vi "Multiple Chassis Synchronization - Scopes Synchronized with TCLK.vi"() -> ()   [LabVIEW 2026]
uses:
  SubVIs/NI SYNC Abstraction/Lib/Trigger Routing.ctl
  SubVIs/NI SYNC Abstraction/Lib/Clock Routing.ctl
  <instrlib>/niScope/Controls/niScope export destinations.ctl
  Types/State.WithTclk.ctl
  <instrlib>/niScope/Controls/niScope input clock source.ctl
  Types/MyVariables.ctl
  <instrlib>/niScope/Controls/niScope exportable signals.ctl
  <instrlib>/niFgen/niFgen.llb/niFgen Output Mode.ctl
  <instrlib>/niScope/Configure/Trigger/niScope Configure Trigger Edge.vi
  <instrlib>/niScope/Configure/Trigger/niScope Configure Trigger Digital.vi
  SubVIs/NI SYNC Abstraction/Lib/Connect Clock Terminals-Array.vi
  SubVIs/NI SYNC Abstraction/Lib/Connect Clock Terminals.vi
  SubVIs/NI SYNC Abstraction/Lib/Connect Trigger Terminals.vi
  SubVIs/NI SYNC Abstraction/Lib/Disonnect Trigger Terminals-Array.vi
  SubVIs/NI SYNC Abstraction/Lib/Disonnect Trigger Terminals.vi
  <instrlib>/niScope/Acquire/Fetch/niScope Fetch Cluster.vi
  SubVIs/NI SYNC Abstraction/Lib/Disconnect Clock Terminals-Array.vi
  SubVIs/NI SYNC Abstraction/Lib/Disconnect Clock Terminals.vi
  <resource>/objmgr/sessionReference.rc
  <vilib>/ptbypt/NI_PtbyPt.lvlib
  <instrlib>/niSync/niSync.llb/niSync Initialize (IVI).vi
  SubVIs/NI SYNC Abstraction/Lib/Connect Trigger Terminals-Array.vi
panel:
  in  "Tab Control":T1(tab)
  in  "Master.Scope":refnum<k15>="PXI1_SCOPE1"
  in  "Rest.Scopes":refnum<k15>[](array[refnum])=["PXI2_SCOPE2"]
  in  "Master.6674T_1":refnum<k15>="PXI1_MasterSync"
  in  "Rest.6674T_1":refnum<k15>="PXI2_RestSync"
  in  "FGEN.Ref":refnum<k15>="PXI1_FGEN1"
  in  "Routing":T2(tab)
  in  "Rest.In --> Clk10":T3={"Source Terminal"="ClkIn", "Destination Terminal"="PXI_Clk10_In"}
  in  "Master.In --> Clk10":T3={"Source Terminal"="ClkIn", "Destination Terminal"="PXI_Clk10_In"}
  in  "Master.Clock --> Out":T3={"Source Terminal"="Oscillator", "Destination Terminal"="ClkOut"}
  in  "Rest.PFI --> Ref Trigger":T4={"Source"="PFI0", "Destination"="PXI_Trig0", "Synchronization Clock"="SyncClkAsync"}
  in  "Master.Ref Trigger --> PFI":T4={"Source"="PXI_Trig0", "Destination"="PFI0", "Synchronization Clock"="SyncClkAsync"}
  in  "Master.Ref Trigger Export":T5="VAL_RTSI_0"
  in  "Rest.Ref Trigger Source":T5="VAL_RTSI_0"
  in  "Rest.Start Trigger Source":T5="VAL_RTSI_1"
  in  "Rest.PFI --> Start Trigger":T4={"Source"="PFI1", "Destination"="PXI_Trig1", "Synchronization Clock"="SyncClkAsync"}
  in  "Master.Start Trigger --> PFI":T4={"Source"="PXI_Trig1", "Destination"="PFI2", "Synchronization Clock"="SyncClkAsync"}
  in  "Master.Start Trigger Export":T5="VAL_RTSI_1"
  in  "Rest.Sync Pulse Source":string(combo)="PXI_Trig2"
  in  "Rest.PFI --> Sync Pulse Source":T4={"Source"="PFI1", "Destination"="PXI_Trig2", "Synchronization Clock"="SyncClkAsync"}
  in  "Master.PFI --> Sync Pulse Source":T4={"Source"="PFI1", "Destination"="PXI_Trig2", "Synchronization Clock"="SyncClkAsync"}
  in  "Master.Sync Pulse Export --> PFI":T4={"Source"="PXI_Trig3", "Destination"="PFI2", "Synchronization Clock"="SyncClkFullSpeed"}
  in  "Master.Sync Pulse Export":string(combo)="PXI_Trig3"
  in  "Master.Sync Pulse Source":string(combo)="PXI_Trig2"
  in  "Enable Cal?":bool
  in  "Calibration Iterations":i32=10
  in  "Master Scope tCLK Delay":dbl format="%#_13p"
  out "Cal Iteration Delays":dbl[](array[numeric]) format="%#_p"
  out "Average Delay":dbl format="%.5p"
  out "Standard Deviation":dbl format="%0.2p"
  out "Waveform Graph":T6(graph)
  out "Sample Offset":dbl
  out "error out":errorcluster
  out "Offset Time (s)":dbl format="%#_p"
  # "Scope"
  # "Sync"
  # "Master"
  # "Ref Trigger Export"
  # "Start Trigger Export"
  # "Sync Pulse Source"
  # "Sync Pulse Export"
  # "Sync"
  # "Scope"
  # "Rest"
  # "Ref Trigger Source"
  # "Start Trigger Source"
  # "Sync Pulse Source"
  # "None"
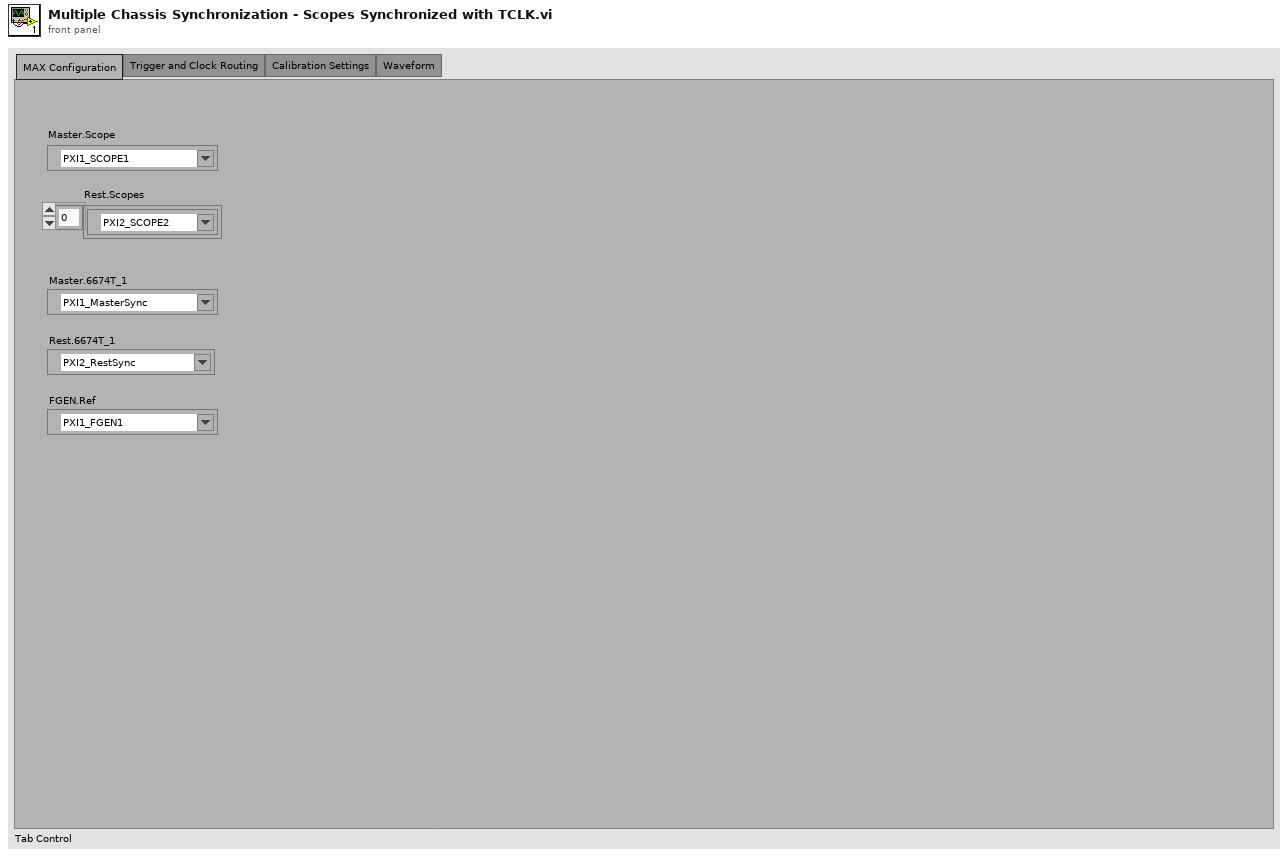
[diagram p1: front panel]
types:
  T1 = enum32{"MAX Configuration", "Trigger and Clock Routing", "Calibration Settings", "Waveform"}
  T2 = enum32{"Clock Routing", "Reference Trigger", "Start Trigger", "Sync Pulse"}
  T3 = typedef "Clock Routing.ctl" = cluster{"Source Terminal":string, "Destination Terminal":string}
  T4 = typedef "Trigger Routing.ctl" = cluster{"Source":string, "Destination":string, "Synchronization Clock":string}
  T5 = typedef "niScope export destinations.ctl" = string
  T6 = cluster{"relativeInitialX":dbl, "xIncrement":dbl, "wfm":dbl[]}[]
  T7 = typedef "State.WithTclk.ctl" = enum16{"Initialize", "SCOPE: Config.Master", "SCOPE: Config.Rest", "SYNC: Device.Init", "SYNC: ConnectClock.Master", "SYNC: ConnectClock.Rest", "SYNC: ConnectSyncPulse.Master", "SYNC: ConnectSyncPulse.Rest", "SYNC: ConnectRefTrigger.Master", "SYNC: ConnectRefTrigger.Rest", "TCLK: Config.Master", "TCLK: Config.Rest", "TCLK: ApplyManualCalibration", "TCLK: SendSyncPulse", "SYNC: DisconnectSyncPulse.Master", "SYNC: DisconnectSyncPulse.Rest", "SYNC: ConnectStartTrigger.Master", "SYNC: ConnectStartTrigger.Rest", "TCLK: Commit", "FGEN: StartSquareWave", "SCOPE: Acquire", "FGEN: StopSquareWave", "SYNC: DisconnectStartTrigger.Master", "SYNC: DisconnectStartTrigger.Rest", "SYNC: DisconnectRefTrigger.Master", "SYNC: DisconnectRefTrigger.Rest", "SYNC: DisconnectClock.Master", "SYNC: DisconnectClock.Rest", "Shutdown"}
  T8 = typedef "MyVariables.ctl" = cluster{"Master":cluster{"TimeSync.Ref":refnum<k15>, "TCLK.Ref":refnum<k20>, "Clock":cluster{"Clock --> Out":T3, "In --> Clk10":T3}, "Sync Pulse":cluster{"Sync Pulse Export":string, "Sync Pulse Export --> PFI":T4, "PFI --> Sync Pulse Source":T4, "Sync Pulse Source":string}, "Start Trigger":cluster{"Start Trigger Export":T5, "Start Trigger --> PFI":T4}, "Scope.Ref":refnum<k15>, "Ref Trigger":cluster{"Ref Trigger Export":T5, "Ref Trigger --> PFI":T4}}, "Rest":cluster{"TimeSync.Ref":refnum<k15>, "TCLK.Refs":refnum<k20>[], "Clock":cluster{"In --> Clk10":T3}, "Sync Pulse":cluster{"PFI --> Sync Pulse Source":T4, "Sync Pulse Source":string}, "Start Trigger":cluster{"PFI --> Start Trigger":T4, "Start Trigger Source":T5}, "Scope.Refs":refnum<k15>[], "Ref Trigger":cluster{"PFI --> Ref Trigger":T4, "Ref Trigger Source":T5}}, "FGEN.Ref":refnum<k15>}
  T9 = typedef "niScope input clock source.ctl" = u16
  T10 = typedef "niScope exportable signals.ctl" = u16
  T11 = typedef "niFgen Output Mode.ctl" = u32
  T12 = cluster{"relativeInitialX":dbl, "xIncrement":dbl, "wfm":dbl[]}
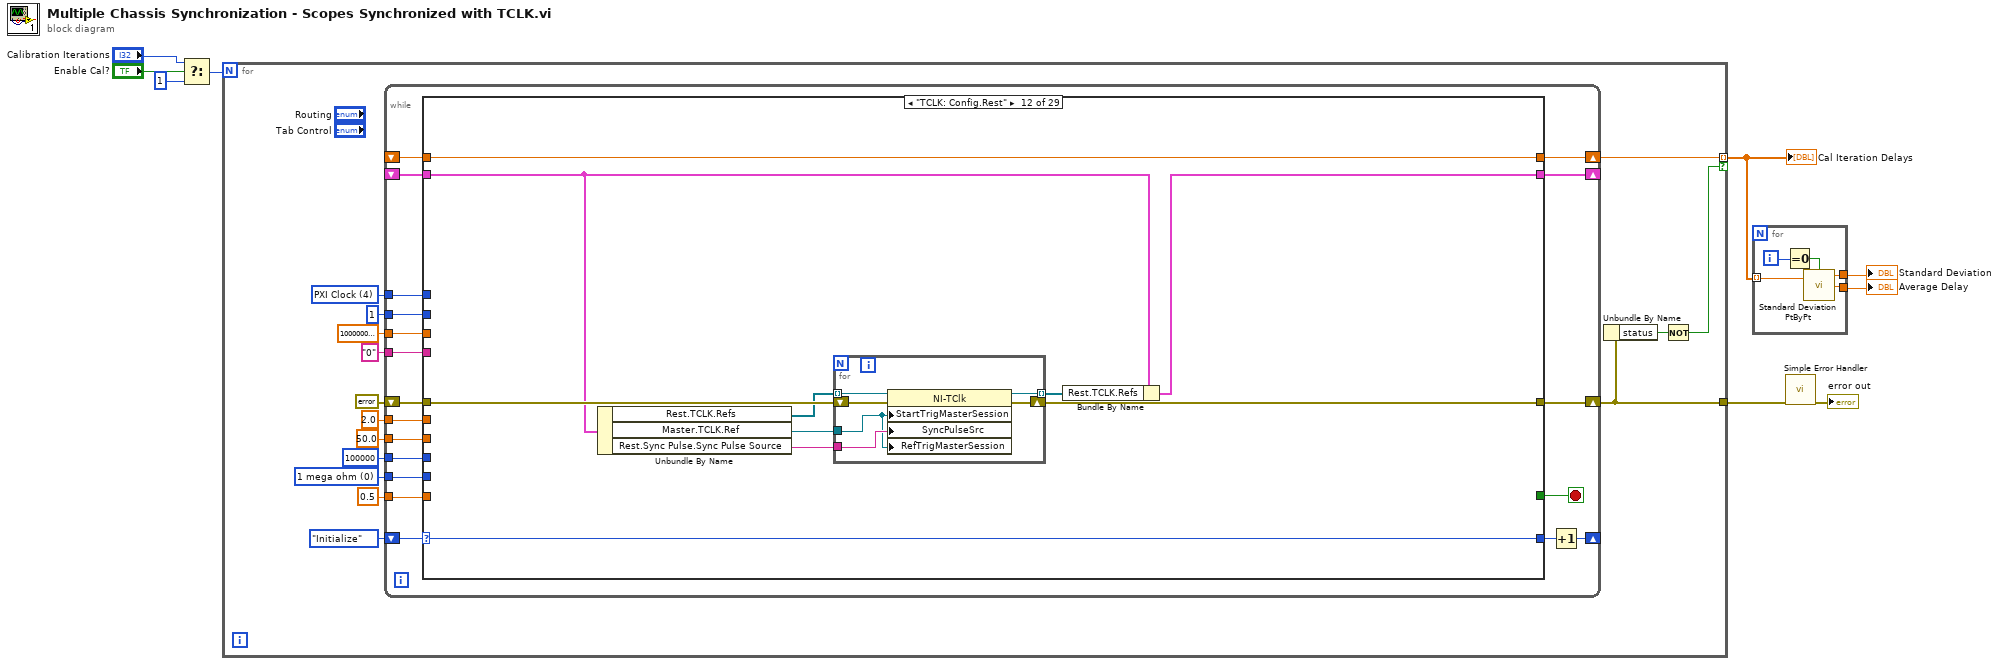
[diagram p0: block diagram]
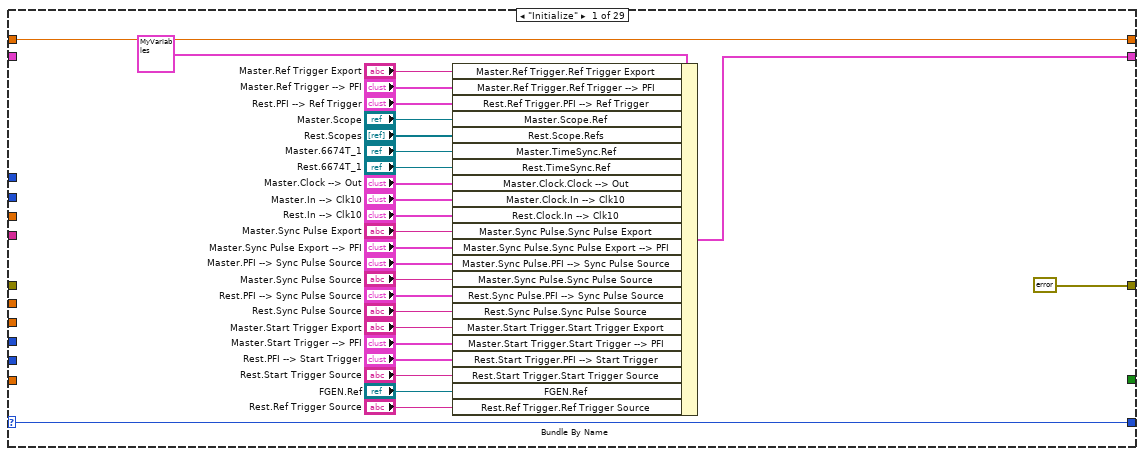
[diagram p2: hidden frame]
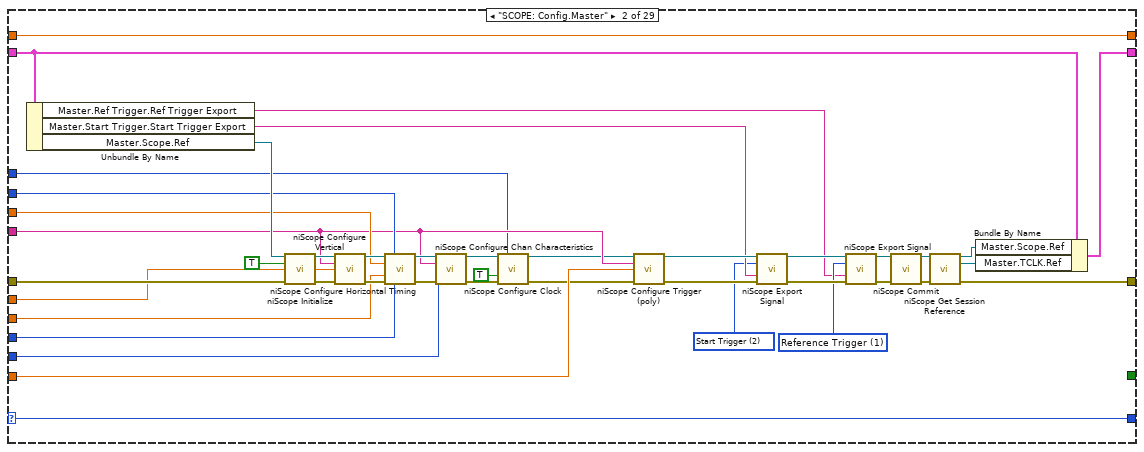
[diagram p3: hidden frame]
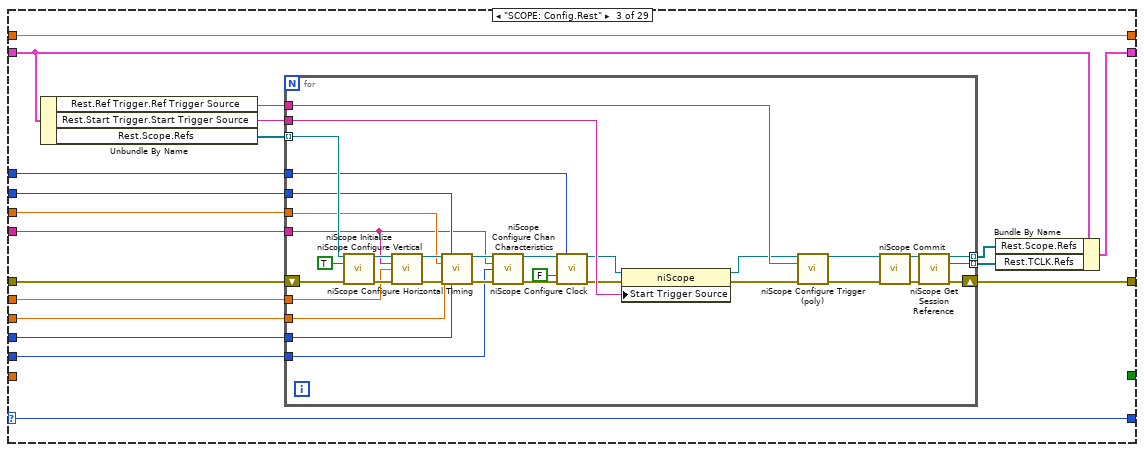
[diagram p4: hidden frame]
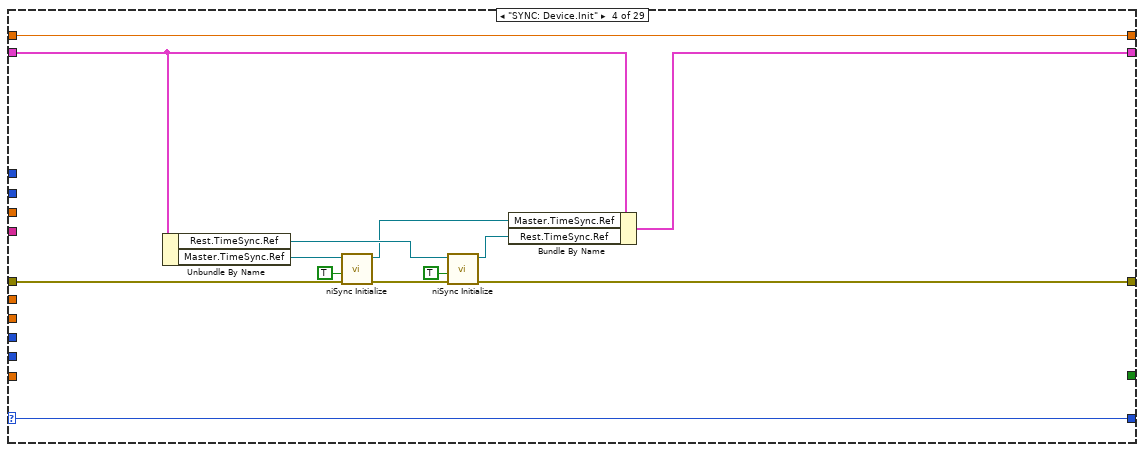
[diagram p5: hidden frame]
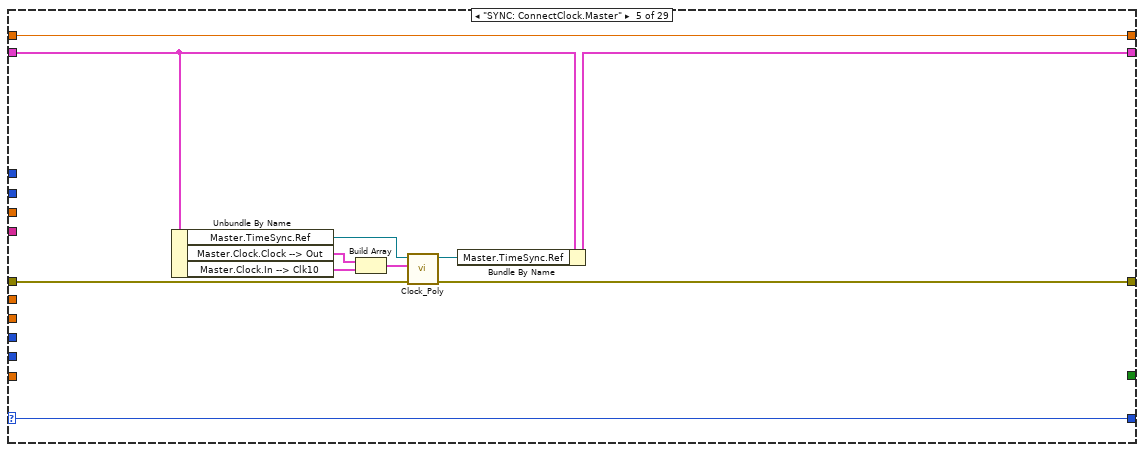
[diagram p6: hidden frame]
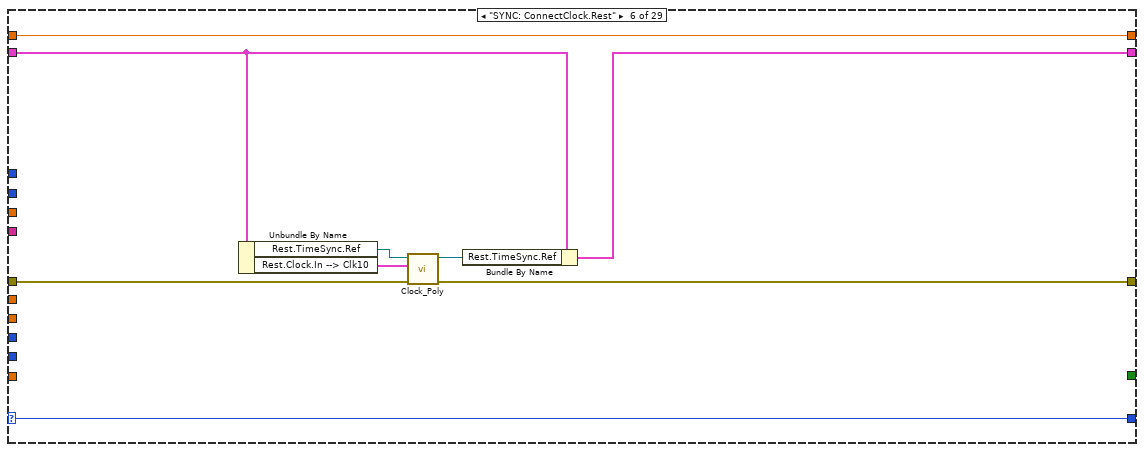
[diagram p7: hidden frame]
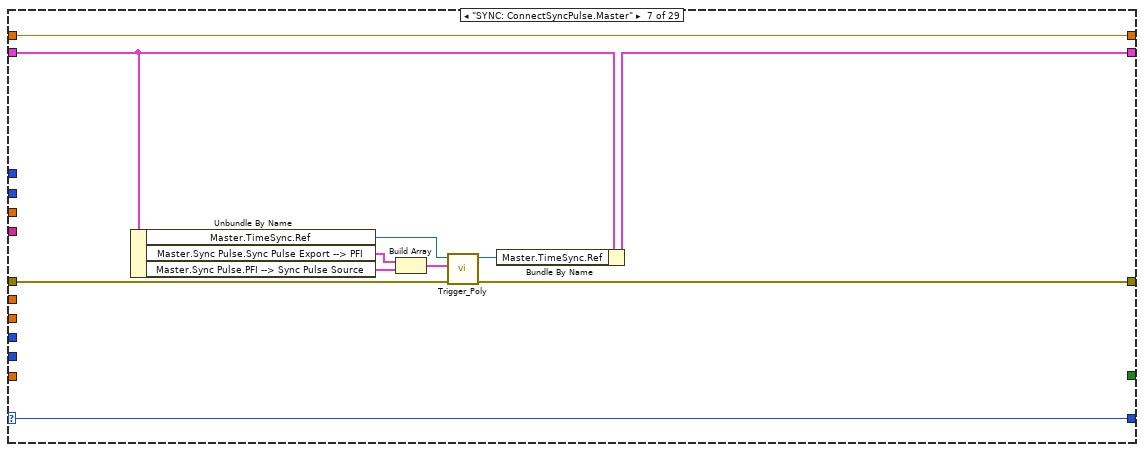
[diagram p8: hidden frame]
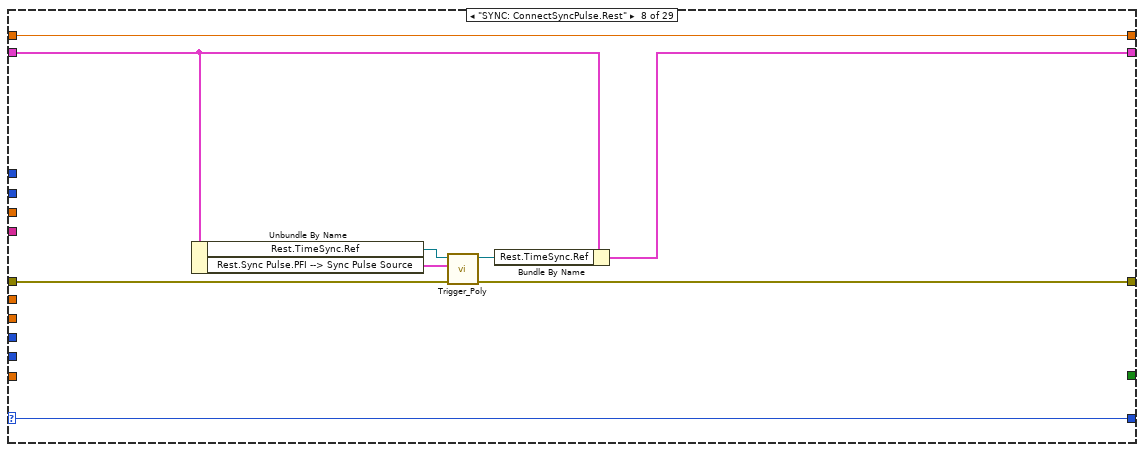
[diagram p9: hidden frame]
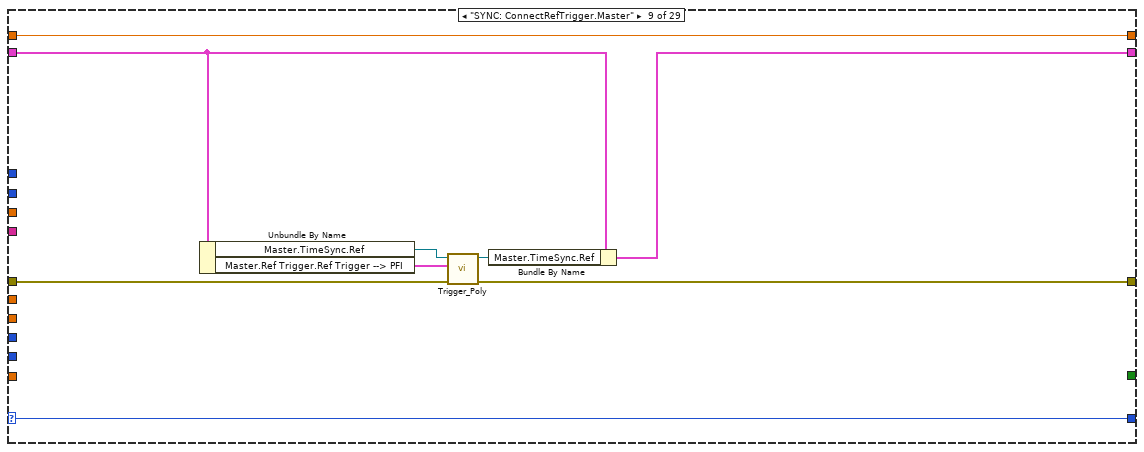
[diagram p10: hidden frame]
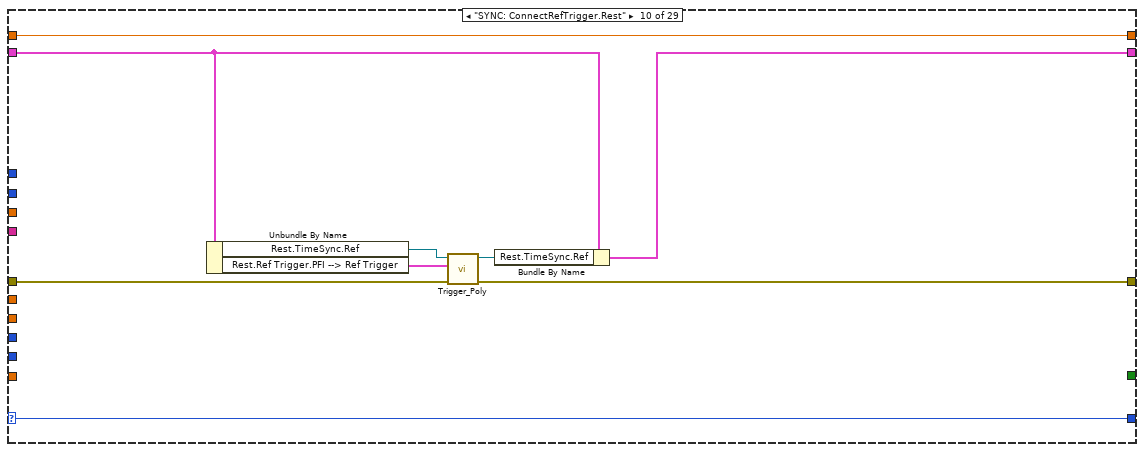
[diagram p11: hidden frame]
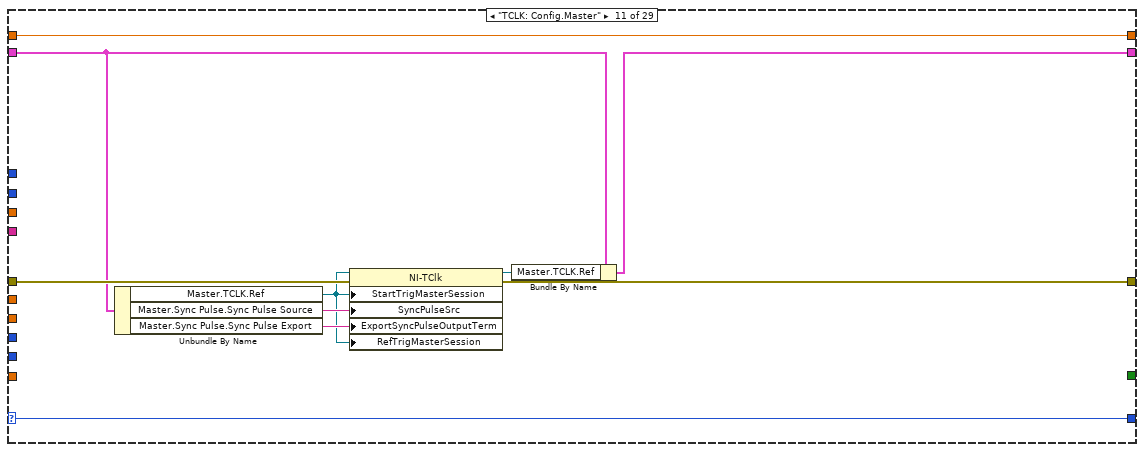
[diagram p12: hidden frame]
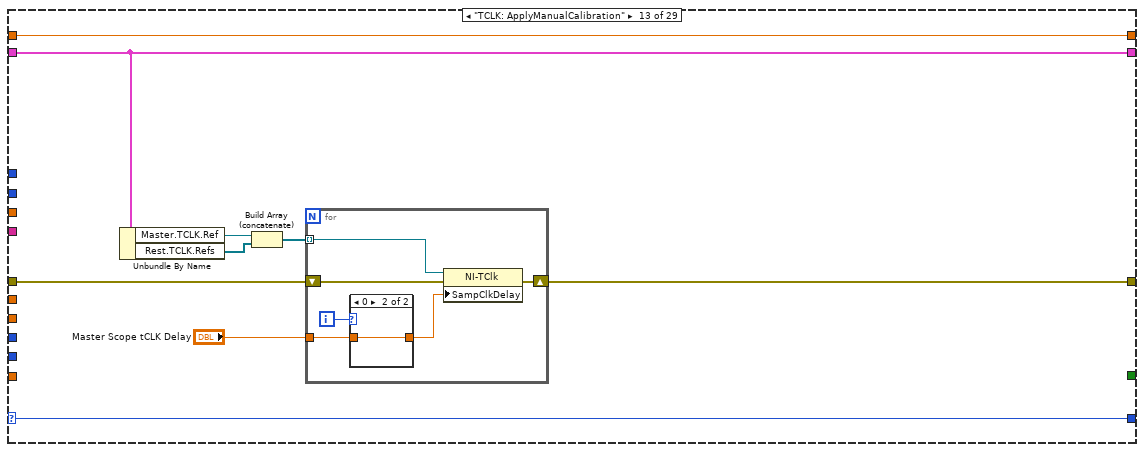
[diagram p13: hidden frame]
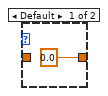
[diagram p14: hidden frame]
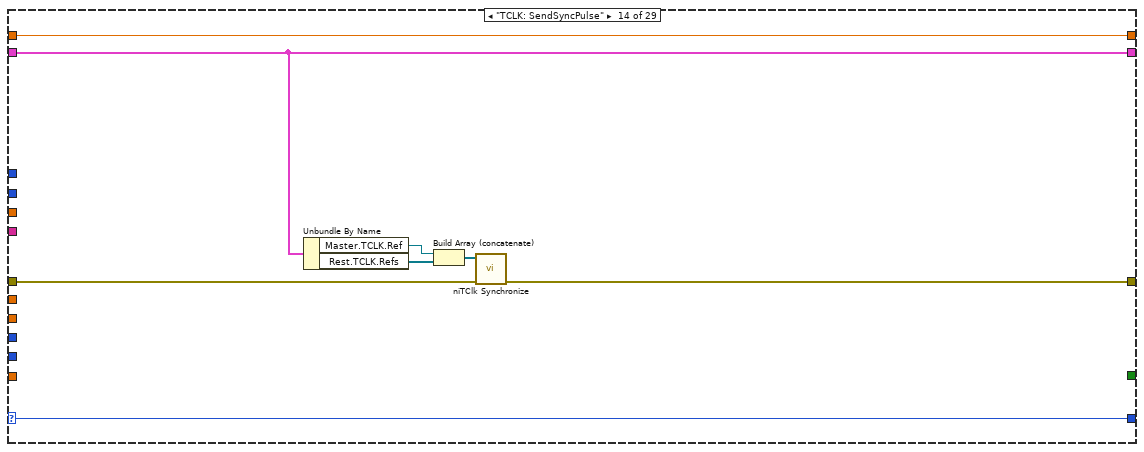
[diagram p15: hidden frame]
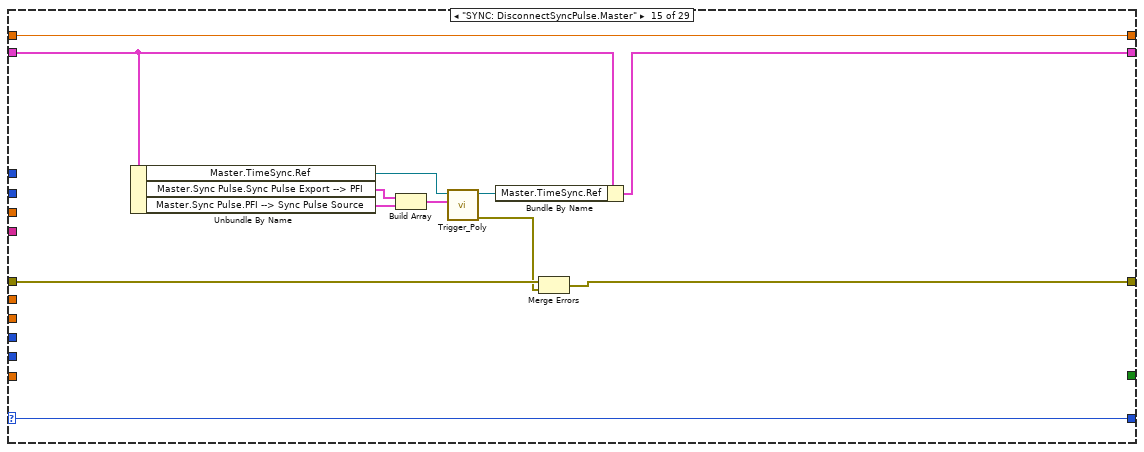
[diagram p16: hidden frame]
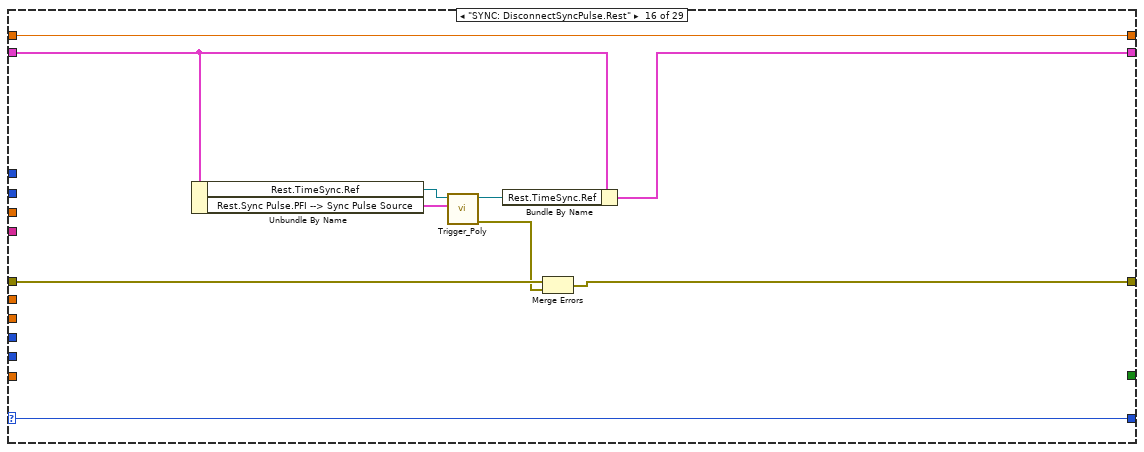
[diagram p17: hidden frame]
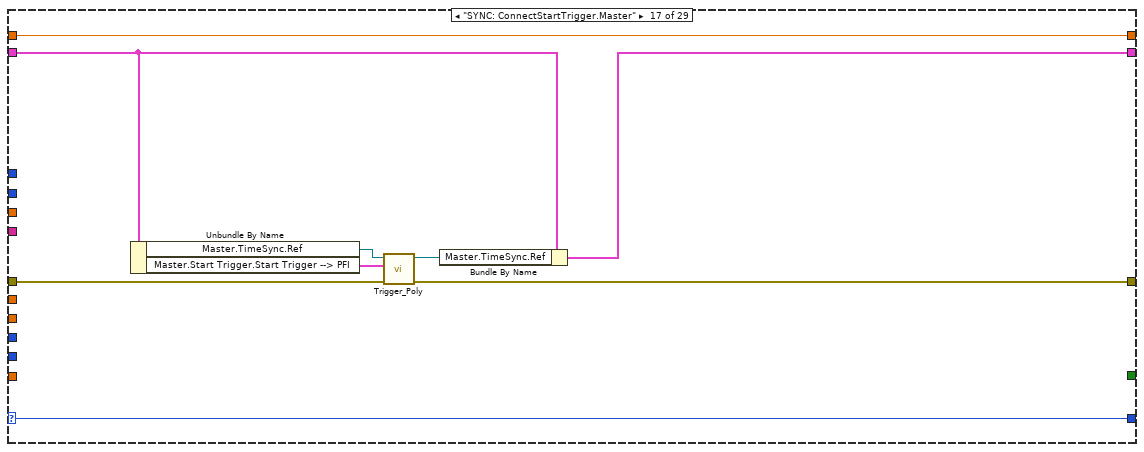
[diagram p18: hidden frame]
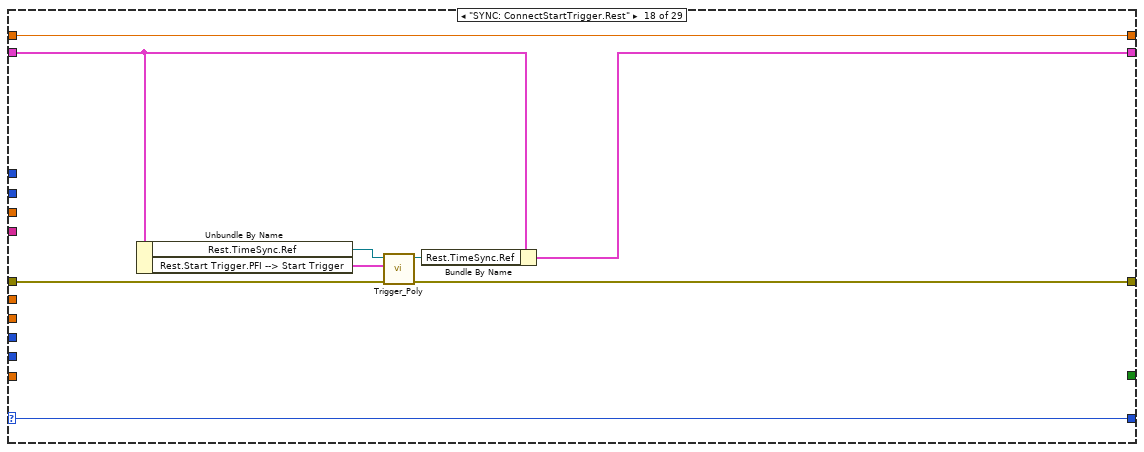
[diagram p19: hidden frame]
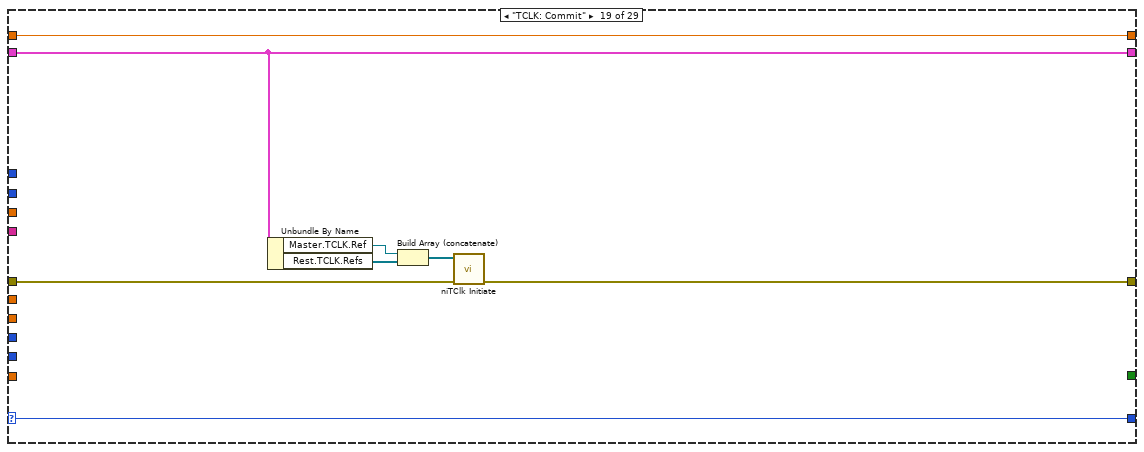
[diagram p20: hidden frame]
diagram:
  n1 = Select(t="Calibration Iterations", s="Enable Cal?", f=1) -> (s? t:f=w4:i32)
  n2 = for {
    N: w4 -> [_]
    tunnel: [w13] -> w9
    tunnel: [w14] -> w3 mode=indexing if=w11
    w10 = T9 4 items=["None"=0, "RTSI Clock"=1, "PFI 0"=6, "PFI 1"=2, "PFI 2"=3, "PXI Clock"=4, "External"=5, "Clock In"=7] ("input clock source")
    w18 = u32 0 items=["1 mega ohm"=0, "50 ohms"=2] ("input impedance")
    n3 = while {
      shift-right: [w36] -> _
      shift-left: State.WithTclk."Initialize" -> [w43]
      shift-right: [w42] -> _
      shift-left: _ -> [w41]
      shift-right: [w39] -> w13
      shift-left: errorcluster {"status"=FALSE, "code"=0, "source"=""} ("error out") -> [w40]
      tunnel: 100000000.0 ("min sample rate") -> [w35]
      tunnel: 100000 ("min record length") -> [w34]
      tunnel: 2.0 ("vertical offset") -> [w33]
      tunnel: 50.0 ("reference position") -> [w32]
      tunnel: w18 -> [w31]
      tunnel: 1 ("number of records") -> [w30]
      tunnel: "0" ("channels") -> [w29]
      tunnel: 0.5 ("trigger level") -> [w28]
      shift-right: [w27] -> w14
      shift-left: _ -> [w26]
      tunnel: w10 -> [w25]
      stop <- w37 stop-if-true
      n4 = case shown="\"TCLK: Config.Rest\"" w43 {
        selector: w43 -> [w53 w112 w131 w167 w179 w191 w199 w211 w220 w229 w245 w255 w270 w286 w291 w304 w311 w320 w334 w344 w376 w388 w400 w411 w421 w431 w440 w453 w460]
        tunnel: [w54 w110 w130 w171 w187 w196 w207 w216 w225 w234 w238 w248 w269 w283 w297 w307 w316 w325 w331 w342 w373 w393 w404 w414 w424 w434 w446 w456 w471] -> w42
        tunnel: w41 -> [_ w96 w127 w172 w188 w197 w208 w217 w226 w235 w240 w250 w269 w283 w298 w308 w317 w326 w331 w336 w373 w393 w405 w415 w425 w435 w447 w457 w471]
        tunnel: [w53 w112 w131 w167 w179 w191 w199 w211 w220 w229 w245 w255 w270 w286 w291 w304 w311 w320 w334 w344 w376 w388 w400 w411 w421 w431 w440 w453 w460] -> w38
        tunnel: [errorcluster {"status"=FALSE, "code"=0, "source"=""} ("error out") w109 w129 w168 w184 w193 w204 w213 w222 w231 w243 w253 w267 w284 w288 w300 w313 w322 w328 w345 w370 w389 w398 w409 w417 w428 w438 w450 w461] -> w39
        tunnel: w40 -> [_ w98 w128 w166 w180 w192 w200 w212 w221 w230 w244 w254 w268 w285 w290 w302 w312 w321 w329 w346 w375 w390 w397 w407 w419 w427 w439 w451 w464]
        tunnel: [_ _ _ _ _ _ _ _ _ _ _ _ _ _ _ _ _ _ _ _ _ _ _ _ _ _ _ _ TRUE] -> w37
        tunnel: w35 -> [_ w84 w120 _ _ _ _ _ _ _ _ _ _ _ _ _ _ _ _ _ w361 _ _ _ _ _ _ _ _]
        tunnel: w34 -> [_ w83 w116 _ _ _ _ _ _ _ _ _ _ _ _ _ _ _ _ _ w362 _ _ _ _ _ _ _ _]
        tunnel: w33 -> [_ w82 w118 _ _ _ _ _ _ _ _ _ _ _ _ _ _ _ _ _ _ _ _ _ _ _ _ _ _]
        tunnel: w32 -> [_ w81 w117 _ _ _ _ _ _ _ _ _ _ _ _ _ _ _ _ _ _ _ _ _ _ _ _ _ _]
        tunnel: w31 -> [_ w80 w115 _ _ _ _ _ _ _ _ _ _ _ _ _ _ _ _ _ _ _ _ _ _ _ _ _ _]
        tunnel: w30 -> [_ w79 w121 _ _ _ _ _ _ _ _ _ _ _ _ _ _ _ _ _ _ _ _ _ _ _ _ _ _]
        tunnel: w29 -> [_ w78 w119 _ _ _ _ _ _ _ _ _ _ _ _ _ _ _ _ _ _ _ _ _ _ _ _ _ _]
        tunnel: w28 -> [_ w77 _ _ _ _ _ _ _ _ _ _ _ _ _ _ _ _ _ w340 w358 _ _ _ _ _ _ _ _]
        tunnel: [w45 w76 w114 w165 w178 w189 w198 w209 w218 w227 w236 w246 w263 w279 w287 w299 w309 w318 w327 w337 w357 w387 w396 w406 w416 w426 w436 w448 w458] -> w27
        tunnel: w26 -> [w45 w76 w114 w165 w178 w189 w198 w209 w218 w227 w236 w246 w263 w279 w287 w299 w309 w318 w327 w337 _ w387 w396 w406 w416 w426 w436 w448 w458]
        tunnel: w25 -> [_ w72 w113 _ _ _ _ _ _ _ _ _ _ _ _ _ _ _ _ _ _ _ _ _ _ _ _ _ _]
        frame "Initialize" {
          n5 = Bundle By Name(cluster=T8 {"Master"={"TimeSync.Ref"="PXI_Trig0", "TCLK.Ref"=refnum, "Clock"={"Clock --> Out"={"Source Terminal"="Oscillator", "Destination Terminal"="ClkOut"}, "In --> Clk10"={"Source Terminal"="ClkIn", "Destination Terminal"="PXI_Clk10_In"}}, "Sync Pulse"={"Sync Pulse Export"="SyncClkFullSpeed", "Sync Pulse Export --> PFI"={"Source"="ClkIn", "Destination"="PXI_Clk10_In", "Synchronization Clock"="SyncClkAsync"}, "PFI --> Sync Pulse Source"={"Source"="PXI_Trig2", "Destination"="PFI2", "Synchronization Clock"="SyncClkAsync"}, "Sync Pulse Source"="PFI1"}, "Start Trigger"={"Start Trigger Export"="PXI_Trig2", "Start Trigger --> PFI"={"Source"="SyncClkAsync", "Destination"="VAL_RTSI_2", "Synchronization Clock"=""}}, "Scope.Ref"="", "Ref Trigger"={"Ref Trigger Export"="VAL_RTSI_2", "Ref Trigger --> PFI"={"Source"="PXI_Trig3", "Destination"="PFI0", "Synchronization Clock"="SyncClkAsync"}}}, "Rest"={"TimeSync.Ref"="", "TCLK.Refs"=[], "Clock"={"In --> Clk10"={"Source Terminal"="PXI_Trig0", "Destination Terminal"="PFI2"}}, "Sync Pulse"={"PFI --> Sync Pulse Source"={"Source"="PFI1", "Destination"="PXI_Trig1", "Synchronization Clock"="SyncClkAsync"}, "Sync Pulse Source"="PXI_Trig1"}, "Start Trigger"={"PFI --> Start Trigger"={"Source"="PFI1", "Destination"="PXI_Trig2", "Synchronization Clock"="SyncClkAsync"}, "Start Trigger Source"="VAL_RTSI_2"}, "Scope.Refs"=[], "Ref Trigger"={"PFI --> Ref Trigger"={"Source"="PFI0", "Destination"="PXI_Trig3", "Synchronization Clock"="SyncClkAsync"}, "Ref Trigger Source"="VAL_RTSI_3"}}, "FGEN.Ref"=""} ("Routes"), "Master.Ref Trigger.Ref Trigger Export"="Master.Ref Trigger Export", "Master.Ref Trigger.Ref Trigger --> PFI"="Master.Ref Trigger --> PFI", "Rest.Ref Trigger.PFI --> Ref Trigger"="Rest.PFI --> Ref Trigger", "Master.Scope.Ref"="Master.Scope", "Rest.Scope.Refs"="Rest.Scopes", "Master.TimeSync.Ref"="Master.6674T_1", "Rest.TimeSync.Ref"="Rest.6674T_1", "Master.Clock.Clock --> Out"="Master.Clock --> Out", "Master.Clock.In --> Clk10"="Master.In --> Clk10", "Rest.Clock.In --> Clk10"="Rest.In --> Clk10", "Master.Sync Pulse.Sync Pulse Export"="Master.Sync Pulse Export", "Master.Sync Pulse.Sync Pulse Export --> PFI"="Master.Sync Pulse Export --> PFI", "Master.Sync Pulse.PFI --> Sync Pulse Source"="Master.PFI --> Sync Pulse Source", "Master.Sync Pulse.Sync Pulse Source"="Master.Sync Pulse Source", "Rest.Sync Pulse.PFI --> Sync Pulse Source"="Rest.PFI --> Sync Pulse Source", "Rest.Sync Pulse.Sync Pulse Source"="Rest.Sync Pulse Source", "Master.Start Trigger.Start Trigger Export"="Master.Start Trigger Export", "Master.Start Trigger.Start Trigger --> PFI"="Master.Start Trigger --> PFI", "Rest.Start Trigger.PFI --> Start Trigger"="Rest.PFI --> Start Trigger", "Rest.Start Trigger.Start Trigger Source"="Rest.Start Trigger Source", "FGEN.Ref"="FGEN.Ref", "Rest.Ref Trigger.Ref Trigger Source"="Rest.Ref Trigger Source") -> (w54:T8)
        }
        frame "SCOPE: Config.Master" {
          w86 = T10 1 items=["None"=0, "Start Trigger"=2, "Advance Trigger"=5, "Reference Trigger"=1, "End of Record Event"=4, "End of Acquisition Event"=3, "Ready for Start Event"=7, "Ready for Advance Event"=6, "Ready for Reference Event"=10, "Reference Clock"=100, "Sample Clock"=101, "5 Volt Power"=13] ("signal")
          w91 = T10 2 items=["None"=0, "Start Trigger"=2, "Advance Trigger"=5, "Reference Trigger"=1, "End of Record Event"=4, "End of Acquisition Event"=3, "Ready for Start Event"=7, "Ready for Advance Event"=6, "Ready for Reference Event"=10, "Reference Clock"=100, "Sample Clock"=101, "5 Volt Power"=13] ("signal")
          n6 = Unbundle By Name(w96) -> ("Master.Ref Trigger.Ref Trigger Export"=w85:T5, "Master.Start Trigger.Start Trigger Export"=w95:T5, "Master.Scope.Ref"=w94:refnum<k15>)
          n7 = call <instrlib>:"niScope Initialize.vi"("resource name"=w94, "id query"=TRUE, "error in"=w98) -> ("instrument handle"=w107:refnum<k15>, "error out"=w104:errorcluster)  [unwired: 11 in]
          n8 = call <instrlib>:"niScope Configure Vertical.vi"("instrument handle"=w107, "channels"=w78, "vertical range"=w82, "error in"=w104) -> ("instrument handle out"=w106:refnum<k15>, "error out"=w103:errorcluster)  [unwired: 10 in]
          n9 = call <instrlib>:"niScope Configure Horizontal Timing.vi"("instrument handle"=w106, "number of records"=w79, "min sample rate"=w84, "reference position"=w81, "error in"=w103, "min record length"=w83) -> ("instrument handle out"=w105:refnum<k15>, "error out"=w102:errorcluster)  [unwired: 8 in]
          n10 = call <instrlib>:"niScope Configure Chan Characteristics.vi"("instrument handle"=w105, "channels"=w78, "input impedance"=w80, "error in"=w102) -> ("instrument handle out"=w101:refnum<k15>, "error out"=w74:errorcluster)  [unwired: 10 in]
          n11 = call <instrlib>:"niScope Configure Clock.vi"("instrument handle"=w101, "input clock source"=w72, "master enabled"=TRUE, "error in"=w74) -> ("instrument handle out"=w75:refnum<k15>, "error out"=w73:errorcluster)  [unwired: 10 in]
          n12 = call-poly <instrlib>:"niScope Configure Trigger (poly).vi"("instrument handle"=w75, "trigger source"=w78, "trigger level"=w77, "error in"=w73) -> ("instrument handle out"=w97:refnum<k15>, "error out"=w100:errorcluster)  [unwired: 10 in]
          n13 = call <instrlib>:"niScope Export Signal.vi"("instrument handle"=w97, "signal"=w91, "output terminal"=w95, "error in"=w100) -> ("instrument handle out"=w89:refnum<k15>, "error out"=w90:errorcluster)  [unwired: 10 in]
          n14 = call <instrlib>:"niScope Export Signal.vi"("instrument handle"=w89, "signal"=w86, "output terminal"=w85, "error in"=w90) -> ("instrument handle out"=w87:refnum<k15>, "error out"=w88:errorcluster)  [unwired: 10 in]
          n15 = call <instrlib>:"niScope Commit.vi"("instrument handle"=w87, "error in"=w88) -> ("instrument handle out"=w93:refnum<k15>, "error out"=w99:errorcluster)  [unwired: 12 in]
          n16 = call <instrlib>:"niScope Get Session Reference.vi"("instrument handle"=w93, "error in"=w99) -> ("instrument handle out"=w92:refnum<k15>, "session reference"=w111:refnum<k20>, "error out"=w109:errorcluster)  [unwired: 11 in]
          n17 = Bundle By Name(cluster=w96, "Master.Scope.Ref"=w92, "Master.TCLK.Ref"=w111) -> (w110:T8)
        }
        frame "SCOPE: Config.Rest" {
          n18 = Unbundle By Name(w127) -> ("Rest.Ref Trigger.Ref Trigger Source"=w122:T5, "Rest.Start Trigger.Start Trigger Source"=w126:T5, "Rest.Scope.Refs"=w123:refnum<k15>[])
          n19 = for {
            tunnel: w126 -> [w154]
            shift-right: [w164] -> w129
            shift-left: w128 -> [w155]
            tunnel: [w150] -> w125 mode=indexing
            tunnel: [w149] -> w124 mode=indexing
            tunnel: w123 -> [w148] mode=indexing
            tunnel: w122 -> [w147]
            tunnel: w121 -> [w144]
            tunnel: w120 -> [w143]
            tunnel: w119 -> [w142]
            tunnel: w118 -> [w141]
            tunnel: w117 -> [w140]
            tunnel: w116 -> [w139]
            tunnel: w115 -> [w138]
            tunnel: w113 -> [w132]
            n20 = call <instrlib>:"niScope Initialize.vi"("resource name"=w148, "id query"=TRUE, "error in"=w155) -> ("instrument handle"=w162:refnum<k15>, "error out"=w159:errorcluster)  [unwired: 11 in]
            n21 = call <instrlib>:"niScope Configure Vertical.vi"("instrument handle"=w162, "channels"=w142, "vertical range"=w141, "error in"=w159) -> ("instrument handle out"=w161:refnum<k15>, "error out"=w158:errorcluster)  [unwired: 10 in]
            n22 = call <instrlib>:"niScope Configure Horizontal Timing.vi"("instrument handle"=w161, "number of records"=w144, "min sample rate"=w143, "reference position"=w140, "error in"=w158, "min record length"=w139) -> ("instrument handle out"=w160:refnum<k15>, "error out"=w157:errorcluster)  [unwired: 8 in]
            n23 = call <instrlib>:"niScope Configure Chan Characteristics.vi"("instrument handle"=w160, "channels"=w142, "input impedance"=w138, "error in"=w157) -> ("instrument handle out"=w136:refnum<k15>, "error out"=w135:errorcluster)  [unwired: 10 in]
            n24 = call <instrlib>:"niScope Configure Clock.vi"("instrument handle"=w136, "input clock source"=w132, "master enabled"=FALSE, "error in"=w135) -> ("instrument handle out"=w133:refnum<k15>, "error out"=w134:errorcluster)  [unwired: 10 in]
            n25 = property class="niScope"(reference=w133, error in=w134, "Start Trigger Source"=w154) -> (reference out=w145:refnum<k15>, error out=w146:errorcluster)
            n26 = call-poly <instrlib>:"niScope Configure Trigger (poly).vi"("instrument handle"=w145, "trigger source"=w147, "error in"=w146) -> ("instrument handle out"=w152:refnum<k15>, "error out"=w153:errorcluster)  [unwired: 11 in]
            n27 = call <instrlib>:"niScope Commit.vi"("instrument handle"=w152, "error in"=w153) -> ("instrument handle out"=w151:refnum<k15>, "error out"=w156:errorcluster)  [unwired: 12 in]
            n28 = call <instrlib>:"niScope Get Session Reference.vi"("instrument handle"=w151, "error in"=w156) -> ("instrument handle out"=w149:refnum<k15>, "session reference"=w150:refnum<k20>, "error out"=w164:errorcluster)  [unwired: 11 in]
          }
          n29 = Bundle By Name(cluster=w127, "Rest.Scope.Refs"=w124, "Rest.TCLK.Refs"=w125) -> (w130:T8)
        }
        frame "SYNC: Device.Init" {
          n30 = Unbundle By Name(w172) -> ("Rest.TimeSync.Ref"=w176:refnum<k15>, "Master.TimeSync.Ref"=w177:refnum<k15>)
          n31 = call-poly <instrlib>:"niSync Initialize.vi"("error in (no error)"=w166, "reset device (F)"=TRUE, "resource name"=w177) -> ("error out"=w175:errorcluster, "instrument handle out"=w170:refnum<k15>)  [unwired: 7 in]
          n32 = call-poly <instrlib>:"niSync Initialize.vi"("error in (no error)"=w175, "reset device (F)"=TRUE, "resource name"=w176) -> ("error out"=w168:errorcluster, "instrument handle out"=w169:refnum<k15>)  [unwired: 7 in]
          n33 = Bundle By Name(cluster=w172, "Master.TimeSync.Ref"=w170, "Rest.TimeSync.Ref"=w169) -> (w171:T8)
        }
        frame "SYNC: ConnectClock.Master" {
          n34 = Unbundle By Name(w188) -> ("Master.TimeSync.Ref"=w186:refnum<k15>, "Master.Clock.Clock --> Out"=w183:T3, "Master.Clock.In --> Clk10"=w182:T3)
          n35 = Build Array(w183, w182) -> (w181:T3[])
          n36 = call-poly "Clock_Poly.vi"("error in (no error)"=w180, "Clock Routing"=w181, "instrument handle"=w186) -> ("error out"=w184:errorcluster, "instrument handle out"=w185:refnum<k15>)  [unwired: 7 in]
          n37 = Bundle By Name(cluster=w188, "Master.TimeSync.Ref"=w185) -> (w187:T8)
        }
        frame "SYNC: ConnectClock.Rest" {
          n38 = Unbundle By Name(w197) -> ("Rest.TimeSync.Ref"=w195:refnum<k15>, "Rest.Clock.In --> Clk10"=w190:T3)
          n39 = call-poly "Clock_Poly.vi"("error in (no error)"=w192, "Clock Routing"=w190, "instrument handle"=w195) -> ("error out"=w193:errorcluster, "instrument handle out"=w194:refnum<k15>)  [unwired: 7 in]
          n40 = Bundle By Name(cluster=w197, "Rest.TimeSync.Ref"=w194) -> (w196:T8)
        }
        frame "SYNC: ConnectSyncPulse.Master" {
          n41 = Unbundle By Name(w208) -> ("Master.TimeSync.Ref"=w206:refnum<k15>, "Master.Sync Pulse.Sync Pulse Export --> PFI"=w203:T4, "Master.Sync Pulse.PFI --> Sync Pulse Source"=w202:T4)
          n42 = Build Array(w203, w202) -> (w201:T4[])
          n43 = call-poly "Trigger_Poly.vi"("error in (no error)"=w200, "Routing Information"=w201, "instrument handle"=w206) -> ("error out"=w204:errorcluster, "instrument handle out"=w205:refnum<k15>)  [unwired: 7 in]
          n44 = Bundle By Name(cluster=w208, "Master.TimeSync.Ref"=w205) -> (w207:T8)
        }
        frame "SYNC: ConnectSyncPulse.Rest" {
          n45 = Unbundle By Name(w217) -> ("Rest.TimeSync.Ref"=w215:refnum<k15>, "Rest.Sync Pulse.PFI --> Sync Pulse Source"=w210:T4)
          n46 = call-poly "Trigger_Poly.vi"("error in (no error)"=w212, "Routing Information"=w210, "instrument handle"=w215) -> ("error out"=w213:errorcluster, "instrument handle out"=w214:refnum<k15>)  [unwired: 7 in]
          n47 = Bundle By Name(cluster=w217, "Rest.TimeSync.Ref"=w214) -> (w216:T8)
        }
        frame "SYNC: ConnectRefTrigger.Master" {
          n48 = Unbundle By Name(w226) -> ("Master.TimeSync.Ref"=w224:refnum<k15>, "Master.Ref Trigger.Ref Trigger --> PFI"=w219:T4)
          n49 = call-poly "Trigger_Poly.vi"("error in (no error)"=w221, "Routing Information"=w219, "instrument handle"=w224) -> ("error out"=w222:errorcluster, "instrument handle out"=w223:refnum<k15>)  [unwired: 7 in]
          n50 = Bundle By Name(cluster=w226, "Master.TimeSync.Ref"=w223) -> (w225:T8)
        }
        frame "SYNC: ConnectRefTrigger.Rest" {
          n51 = Unbundle By Name(w235) -> ("Rest.TimeSync.Ref"=w233:refnum<k15>, "Rest.Ref Trigger.PFI --> Ref Trigger"=w228:T4)
          n52 = call-poly "Trigger_Poly.vi"("error in (no error)"=w230, "Routing Information"=w228, "instrument handle"=w233) -> ("error out"=w231:errorcluster, "instrument handle out"=w232:refnum<k15>)  [unwired: 7 in]
          n53 = Bundle By Name(cluster=w235, "Rest.TimeSync.Ref"=w232) -> (w234:T8)
        }
        frame "TCLK: Config.Master" {
          n54 = Unbundle By Name(w240) -> ("Master.TCLK.Ref"=w237:refnum<k20>, "Master.Sync Pulse.Sync Pulse Source"=w242:string, "Master.Sync Pulse.Sync Pulse Export"=w241:string)
          n55 = property class="NI-TClk"(reference=w237, error in=w244, "StartTrigMasterSession"=w237, "SyncPulseSrc"=w242, "ExportSyncPulseOutputTerm"=w241, "RefTrigMasterSession"=w237) -> (reference out=w239:refnum<k20>, error out=w243:errorcluster)
          n56 = Bundle By Name(cluster=w240, "Master.TCLK.Ref"=w239) -> (w238:T8)
        }
        frame "TCLK: Config.Rest" {
          n57 = Unbundle By Name(w250) -> ("Rest.TCLK.Refs"=w252:refnum<k20>[], "Master.TCLK.Ref"=w247:refnum<k20>, "Rest.Sync Pulse.Sync Pulse Source"=w251:string)
          n58 = for {
            tunnel: w252 -> [w259] mode=indexing
            tunnel: w251 -> [w258]
            tunnel: [w257] -> w249 mode=indexing
            tunnel: w247 -> [w256]
            shift-right: [w260] -> w253
            shift-left: w254 -> [w261]
            n59 = property class="NI-TClk"(reference=w259, error in=w261, "StartTrigMasterSession"=w256, "SyncPulseSrc"=w258, "RefTrigMasterSession"=w256) -> (reference out=w257:refnum<k20>, error out=w260:errorcluster)
          }
          n60 = Bundle By Name(cluster=w250, "Rest.TCLK.Refs"=w249) -> (w248:T8)
        }
        frame "TCLK: ApplyManualCalibration" {
          n61 = Unbundle By Name(w269) -> ("Master.TCLK.Ref"=w266:refnum<k20>, "Rest.TCLK.Refs"=w265:refnum<k20>[])
          n62 = Build Array (concatenate)(w266, w265) -> (w264:refnum<k20>[])
          n63 = for {
            shift-right: [w274] -> w267
            shift-left: w268 -> [w275]
            tunnel: w264 -> [w272] mode=indexing
            tunnel: "Master Scope tCLK Delay" -> [w271]
            i -> [w276]
            n64 = case shown="0" w276 {
              tunnel: [0.0 ("delay") w278] -> w273
              tunnel: w271 -> [_ w278]
              frame Default {
              }
              frame 0 {
              }
            }
            n65 = property class="NI-TClk"(reference=w272, error in=w275, "SampClkDelay"=w273) -> (error out=w274:errorcluster)  [unwired: 1 out]
          }
        }
        frame "TCLK: SendSyncPulse" {
          n66 = Unbundle By Name(w283) -> ("Master.TCLK.Ref"=w282:refnum<k20>, "Rest.TCLK.Refs"=w281:refnum<k20>[])
          n67 = Build Array (concatenate)(w282, w281) -> (w280:refnum<k20>[])
          n68 = call <instrlib>:"niTClk Synchronize.vi"("error in (no error)"=w285, "sessions"=w280) -> ("error out"=w284:errorcluster)  [unwired: 8 in, 1 out]
        }
        frame "SYNC: DisconnectSyncPulse.Master" {
          n69 = Unbundle By Name(w298) -> ("Master.TimeSync.Ref"=w296:refnum<k15>, "Master.Sync Pulse.Sync Pulse Export --> PFI"=w294:T4, "Master.Sync Pulse.PFI --> Sync Pulse Source"=w293:T4)
          n70 = Build Array(w294, w293) -> (w292:T4[])
          n71 = call-poly "Trigger_Poly.vi"("Routing Information"=w292, "instrument handle"=w296) -> ("error out"=w289:errorcluster, "instrument handle out"=w295:refnum<k15>)  [unwired: 8 in]
          n72 = Bundle By Name(cluster=w298, "Master.TimeSync.Ref"=w295) -> (w297:T8)
          n73 = Merge Errors(w290, w289) -> (w288:errorcluster)
        }
        frame "SYNC: DisconnectSyncPulse.Rest" {
          n74 = Unbundle By Name(w308) -> ("Rest.TimeSync.Ref"=w306:refnum<k15>, "Rest.Sync Pulse.PFI --> Sync Pulse Source"=w303:T4)
          n75 = call-poly "Trigger_Poly.vi"("Routing Information"=w303, "instrument handle"=w306) -> ("error out"=w301:errorcluster, "instrument handle out"=w305:refnum<k15>)  [unwired: 8 in]
          n76 = Bundle By Name(cluster=w308, "Rest.TimeSync.Ref"=w305) -> (w307:T8)
          n77 = Merge Errors(w302, w301) -> (w300:errorcluster)
        }
        frame "SYNC: ConnectStartTrigger.Master" {
          n78 = Unbundle By Name(w317) -> ("Master.TimeSync.Ref"=w315:refnum<k15>, "Master.Start Trigger.Start Trigger --> PFI"=w310:T4)
          n79 = call-poly "Trigger_Poly.vi"("error in (no error)"=w312, "Routing Information"=w310, "instrument handle"=w315) -> ("error out"=w313:errorcluster, "instrument handle out"=w314:refnum<k15>)  [unwired: 7 in]
          n80 = Bundle By Name(cluster=w317, "Master.TimeSync.Ref"=w314) -> (w316:T8)
        }
        frame "SYNC: ConnectStartTrigger.Rest" {
          n81 = Unbundle By Name(w326) -> ("Rest.TimeSync.Ref"=w324:refnum<k15>, "Rest.Start Trigger.PFI --> Start Trigger"=w319:T4)
          n82 = call-poly "Trigger_Poly.vi"("error in (no error)"=w321, "Routing Information"=w319, "instrument handle"=w324) -> ("error out"=w322:errorcluster, "instrument handle out"=w323:refnum<k15>)  [unwired: 7 in]
          n83 = Bundle By Name(cluster=w326, "Rest.TimeSync.Ref"=w323) -> (w325:T8)
        }
        frame "TCLK: Commit" {
          n84 = Unbundle By Name(w331) -> ("Master.TCLK.Ref"=w333:refnum<k20>, "Rest.TCLK.Refs"=w332:refnum<k20>[])
          n85 = Build Array (concatenate)(w333, w332) -> (w330:refnum<k20>[])
          n86 = call <instrlib>:"niTClk Initiate.vi"("error in (no error)"=w329, "sessions"=w330) -> ("error out"=w328:errorcluster)  [unwired: 8 in, 1 out]
        }
        frame "FGEN: StartSquareWave" {
          w349 = u16 1 items=["Sine", "Square", "Triangle", "Ramp Up", "Ramp Down", "DC", "Noise"] ("Standard Waveform")
          w347 = T11 0 items=["Standard Function", "Frequency List", "Arbitrary Waveform", "Arbitrary Sequence", "Script"] ("output mode")
          n87 = Unbundle By Name(w336) -> ("FGEN.Ref"=w335:refnum<k15>)
          n88 = Multiply(x=2.0, y=w340) -> (x*y=w339:dbl)
          n89 = call <instrlib>:"niFgen Initialize With Channels.vi"("error in (no error)"=w346, "Reset Device (default: False)"=TRUE, "Channel Name"="0", "Resource Name"=w335) -> ("error out"=w356:errorcluster, "Instrument Handle Out"=w355:refnum<k15>)  [unwired: 6 in]
          n90 = call <instrlib>:"niFgen Configure Output Mode.vi"("error in (no error)"=w356, "Output Mode (default: 0=Standard Function)"=w347, "Instrument Handle"=w355) -> ("error out"=w354:errorcluster, "Instrument Handle Out"=w353:refnum<k15>)  [unwired: 6 in]
          n91 = call <instrlib>:"niFgen Configure Standard Waveform.vi"("Instrument Handle"=w353, "Waveform"=w349, "Frequency"=10000.0, "Amplitude"=w339, "error in (no error)"=w354) -> ("Instrument Handle Out"=w352:refnum<k15>, "error out"=w351:errorcluster)  [unwired: 9 in]
          n92 = call <instrlib>:"niFgen Initiate Generation.vi"("error in (no error)"=w351, "Instrument Handle"=w352) -> ("error out"=w345:errorcluster, "Instrument Handle Out"=w343:refnum<k15>)  [unwired: 8 in]
          n93 = Bundle By Name(cluster=w336, "FGEN.Ref"=w343) -> (w342:T8)
        }
        frame "SCOPE: Acquire" {
          n94 = Unbundle By Name(w373) -> ("Master.Scope.Ref"=w371:refnum<k15>, "Rest.Scope.Refs"=w372:refnum<k15>[])
          n95 = Build Array (concatenate)(w371, w372) -> (w369:refnum<k15>[])
          n96 = Array Size(array=w369) -> (size(s)=w368:i32)
          n97 = for {
            tunnel: w369 -> [w383] mode=indexing
            tunnel: [w378] -> w363 mode=indexing
            tunnel: w375 -> [w382]
            tunnel: [w386] -> w374 mode=indexing
            workers-P: w368 -> [_]
            tunnel: w362 -> [w377]
            w379 = 477 items=["Start"=482, "Trigger"=483, "Pretrigger"=477, "Now"=481, "Read Pointer"=388] ("Fetch:Fetch Relative To")
            n98 = property class="niScope"(reference=w383, error in=w382, "Fetch:Fetch Relative To"=w379) -> (reference out=w380:refnum<k15>, error out=w381:errorcluster)
            n99 = call-poly <instrlib>:"niScope Fetch (poly).vi"("timeout"=10.0, "error in"=w381, "numSamples"=w377, "channels"="0", "instrument handle"=w380) -> ("error out"=w386:errorcluster, "waveform"=w378:T12)  [unwired: 3 in, 2 out]
          }
          "Waveform Graph" <- w363
          n100 = Reciprocal(x=w361) -> (1/x=w359:dbl)
          n101 = Merge Errors(w374) -> (w370:errorcluster)
          n102 = Index Array(array=w363) -> (element #1=w367:T12, element #2=w366:T12)  [unwired: 2 in]
          n103 = Unbundle By Name(w367) -> ("wfm"=w364:dbl[])
          n104 = Unbundle By Name(w366) -> ("wfm"=w365:dbl[])
          n105 = call "Find Delta Samples of Rising Edge_DBL.vi"("Trigger Level"=w358, "Channel 2"=w365, "Channel 1"=w364) -> ("Sample Offset"=w360:dbl)  [unwired: 8 in]
          "Sample Offset" <- w360
          n106 = Multiply(x=w359, y=w360) -> (x*y=w357:dbl)
          "Offset Time (s)" <- w357
        }
        frame "FGEN: StopSquareWave" {
          n107 = Unbundle By Name(w393) -> ("FGEN.Ref"=w392:refnum<k15>)
          n108 = call <instrlib>:"niFgen Abort Generation.vi"("Instrument Handle"=w392) -> ("error out"=w395:errorcluster, "Instrument Handle Out"=w394:refnum<k15>)  [unwired: 9 in]
          n109 = call <instrlib>:"niFgen Close.vi"("error in (no error)"=w395, "Instrument Handle"=w394) -> ("error out"=w391:errorcluster)  [unwired: 9 in]
          n110 = Merge Errors(w390, w391) -> (w389:errorcluster)
        }
        frame "SYNC: DisconnectStartTrigger.Master" {
          n111 = Unbundle By Name(w405) -> ("Master.TimeSync.Ref"=w403:refnum<k15>, "Master.Start Trigger.Start Trigger --> PFI"=w399:T4)
          n112 = call-poly "Trigger_Poly.vi"("Routing Information"=w399, "instrument handle"=w403) -> ("error out"=w401:errorcluster, "instrument handle out"=w402:refnum<k15>)  [unwired: 8 in]
          n113 = Bundle By Name(cluster=w405, "Master.TimeSync.Ref"=w402) -> (w404:T8)
          n114 = Merge Errors(w397, w401) -> (w398:errorcluster)
        }
        frame "SYNC: DisconnectStartTrigger.Rest" {
          n115 = Unbundle By Name(w415) -> ("Rest.TimeSync.Ref"=w413:refnum<k15>, "Rest.Start Trigger.PFI --> Start Trigger"=w410:T4)
          n116 = call-poly "Trigger_Poly.vi"("Routing Information"=w410, "instrument handle"=w413) -> ("error out"=w408:errorcluster, "instrument handle out"=w412:refnum<k15>)  [unwired: 8 in]
          n117 = Bundle By Name(cluster=w415, "Rest.TimeSync.Ref"=w412) -> (w414:T8)
          n118 = Merge Errors(w407, w408) -> (w409:errorcluster)
        }
        frame "SYNC: DisconnectRefTrigger.Master" {
          n119 = Unbundle By Name(w425) -> ("Master.TimeSync.Ref"=w423:refnum<k15>, "Master.Ref Trigger.Ref Trigger --> PFI"=w420:T4)
          n120 = call-poly "Trigger_Poly.vi"("Routing Information"=w420, "instrument handle"=w423) -> ("error out"=w418:errorcluster, "instrument handle out"=w422:refnum<k15>)  [unwired: 8 in]
          n121 = Bundle By Name(cluster=w425, "Master.TimeSync.Ref"=w422) -> (w424:T8)
          n122 = Merge Errors(w419, w418) -> (w417:errorcluster)
        }
        frame "SYNC: DisconnectRefTrigger.Rest" {
          n123 = Unbundle By Name(w435) -> ("Rest.TimeSync.Ref"=w433:refnum<k15>, "Rest.Ref Trigger.PFI --> Ref Trigger"=w430:T4)
          n124 = call-poly "Trigger_Poly.vi"("Routing Information"=w430, "instrument handle"=w433) -> ("error out"=w429:errorcluster, "instrument handle out"=w432:refnum<k15>)  [unwired: 8 in]
          n125 = Bundle By Name(cluster=w435, "Rest.TimeSync.Ref"=w432) -> (w434:T8)
          n126 = Merge Errors(w427, w429) -> (w428:errorcluster)
        }
        frame "SYNC: DisconnectClock.Master" {
          n127 = Unbundle By Name(w447) -> ("Master.TimeSync.Ref"=w445:refnum<k15>, "Master.Clock.Clock --> Out"=w443:T3, "Master.Clock.In --> Clk10"=w442:T3)
          n128 = Build Array(w443, w442) -> (w441:T3[])
          n129 = call-poly "Clock_Poly.vi"("Clock Routing"=w441, "instrument handle"=w445) -> ("error out"=w437:errorcluster, "instrument handle out"=w444:refnum<k15>)  [unwired: 8 in]
          n130 = Bundle By Name(cluster=w447, "Master.TimeSync.Ref"=w444) -> (w446:T8)
          n131 = Merge Errors(w439, w437) -> (w438:errorcluster)
        }
        frame "SYNC: DisconnectClock.Rest" {
          n132 = Unbundle By Name(w457) -> ("Rest.TimeSync.Ref"=w455:refnum<k15>, "Rest.Clock.In --> Clk10"=w452:T3)
          n133 = call-poly "Clock_Poly.vi"("Clock Routing"=w452, "instrument handle"=w455) -> ("error out"=w449:errorcluster, "instrument handle out"=w454:refnum<k15>)  [unwired: 8 in]
          n134 = Bundle By Name(cluster=w457, "Rest.TimeSync.Ref"=w454) -> (w456:T8)
          n135 = Merge Errors(w451, w449) -> (w450:errorcluster)
        }
        frame "Shutdown" {
          n136 = Unbundle By Name(w471) -> ("Master.TimeSync.Ref"=w470:refnum<k15>, "Rest.TimeSync.Ref"=w469:refnum<k15>, "Master.Scope.Ref"=w468:refnum<k15>, "Rest.Scope.Refs"=w467:refnum<k15>[])
          n137 = Build Array(w470, w469) -> (w465:refnum<k15>[])
          n138 = Build Array (concatenate)(w468, w467) -> (w466:refnum<k15>[])
          n139 = for {
            tunnel: w465 -> [w473] mode=indexing
            tunnel: [w472] -> w462 mode=indexing
            n140 = call <instrlib>:"niSync Close.vi"("instrument handle"=w473) -> ("error out"=w472:errorcluster)  [unwired: 10 in]
          }
          n141 = for {
            tunnel: w466 -> [w475] mode=indexing
            tunnel: [w474] -> w463 mode=indexing
            n142 = call <instrlib>:"niScope Close.vi"("instrument handle"=w475) -> ("error out"=w474:errorcluster)  [unwired: 14 in]
          }
          n143 = Merge Errors(w464, w463, w462) -> (w461:errorcluster)
        }
      }
      n144 = Increment(x=w38) -> (x+1=w36:T7)
    }
    n145 = Unbundle By Name(w13) -> ("status"=w12:bool)
    n146 = Not(x=w12) -> (.not. x?=w11:bool)
  }
  "Cal Iteration Delays" <- w3
  n147 = for {
    tunnel: w3 -> [w480] mode=indexing
    tunnel: [w479] -> w1
    tunnel: [w478] -> w2
    i -> [w477]
    n148 = Equal To 0?(x=w477) -> (x = 0?=w476:bool)
    n149 = call <vilib>:"Standard Deviation PtByPt.vi"("x"=w480, "initialize"=w476) -> ("standard deviation"=w479:dbl, "mean"=w478:dbl)  [unwired: 1 in, 1 out]
  }
  "Average Delay" <- w2
  "Standard Deviation" <- w1
  n150 = call <vilib>:"Simple Error Handler.vi"("error in (no error)"=w9) -> ("error out"=→"error out":errorcluster)  [unwired: 4 in, 4 out]
